vi "Multicolor_line_generator.vi"() -> ()   [LabVIEW 2020]
uses:
  ASLM project/type_defs/Laser_toggles_typedef.ctl
  <vilib>/Utility/file.llb/Read Delimited Spreadsheet (DBL).vi
  <vilib>/measure/NI_MABase.lvlib
panel:
  in  "Laser 642 nm power":dbl(slide) min=0.0 max=5.0 scale=0.0..5.0
  in  "Laser 595 nm power":dbl(slide) min=0.0 max=5.0 scale=0.0..5.0
  in  "Laser 560 nm power":dbl(slide) min=0.0 max=5.0 scale=0.0..5.0
  in  "Laser 488 nm power":dbl(slide) min=0.0 max=5.0 scale=0.0..5.0
  in  "Time for one frame":dbl
  out "Number of active lasers":dbl
  out "Laser Toggles":T1
  in  "Time between acquisitions":dbl
  in  "File to read":path=path "C:/Users/Hannah/Downloads/newcalibration_voice coil input_25msflyback_3075datapoints.txt"
  out "LabVIEW generated Sawtooth input (blue) and Camera trigger (red)":waveform(dbl)[](graph)=[{"t0"=timestamp(0 s since 1904-01-01), "dt"=1.0, "Y"=array[3075 elements]}, {"t0"=timestamp(0 s since 1904-01-01), "dt"=0.001, "Y"=array[3075 elements]}, {"t0"=timestamp(0 s since 1904-01-01), "dt"=0.001, "Y"=array[3075 elements]}, {"t0"=timestamp(0 s since 1904-01-01), "dt"=0.001, "Y"=array[3075 elements]}]
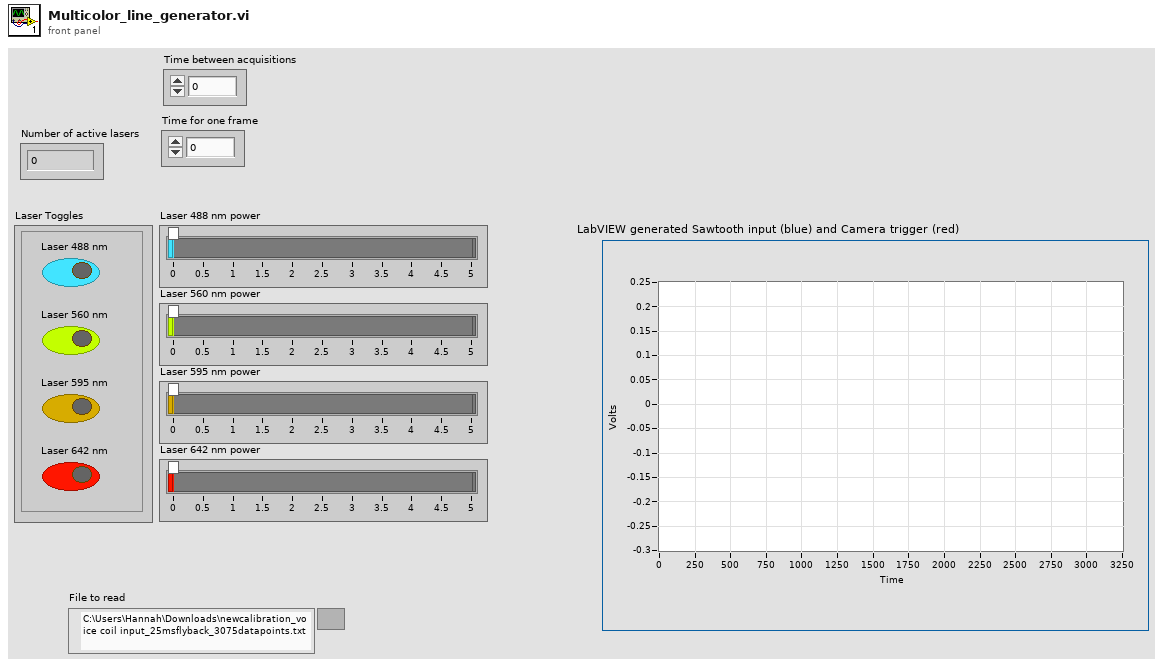
[diagram p1: front panel]
types:
  T1 = typedef "Laser_toggles_typedef.ctl" = cluster{"Laser 488 nm":bool, "Laser 560 nm":bool, "Laser 595 nm":bool, "Laser 642 nm":bool}
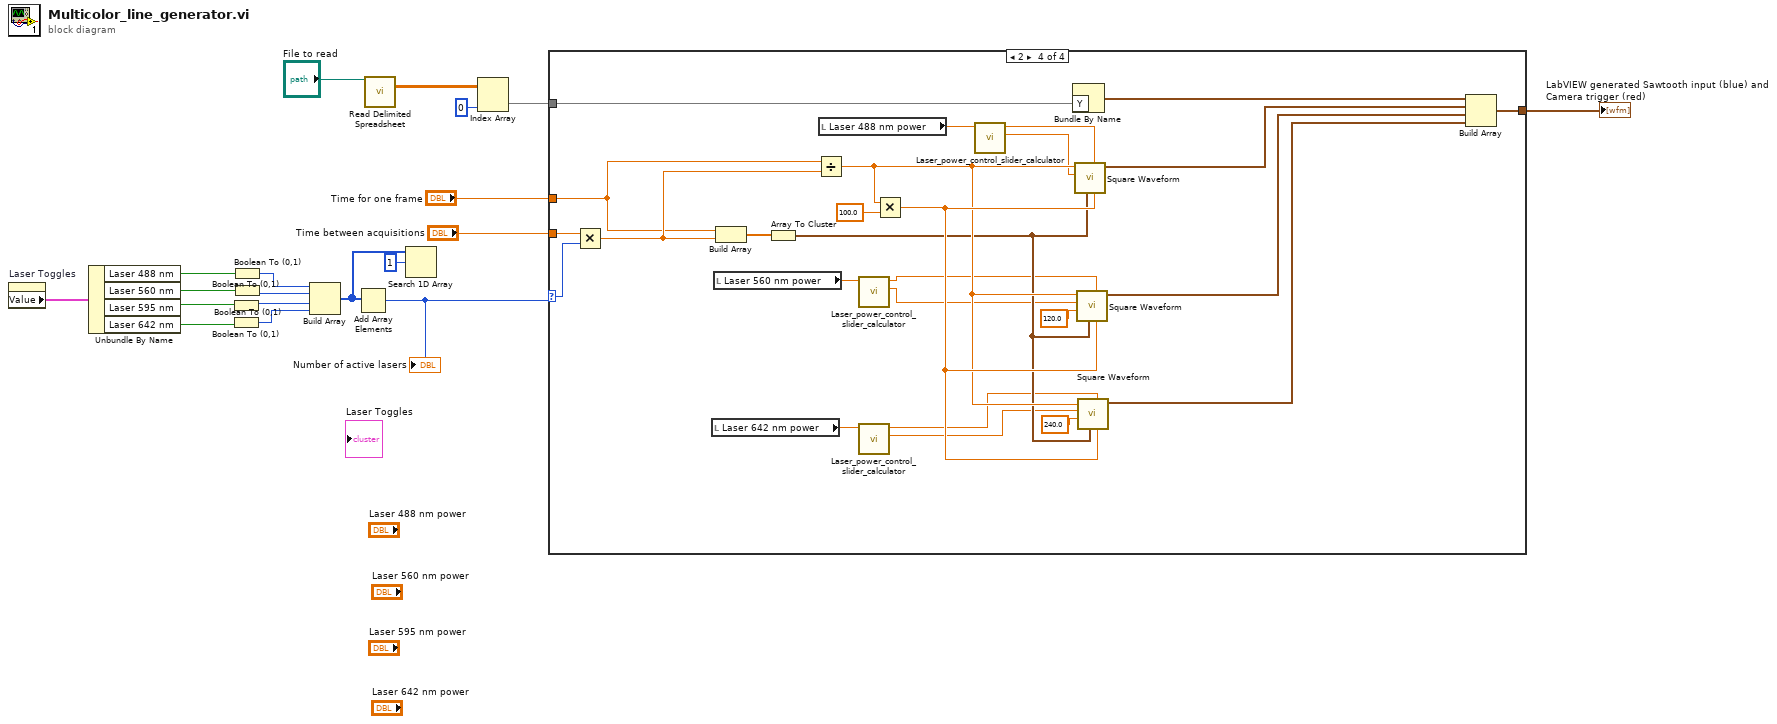
[diagram p0: block diagram]
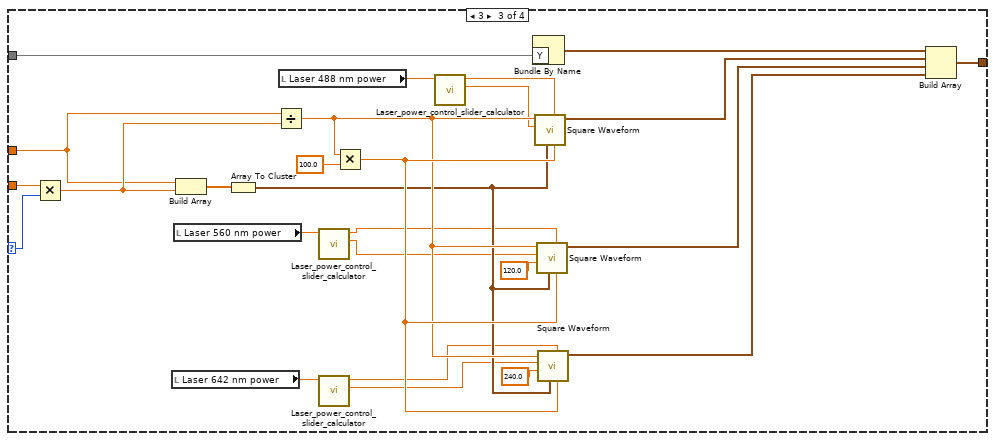
[diagram p4: hidden frame]
diagram:
  n1 = property on="Laser Toggles" class="Clust (strict)"() -> ("Value"=w14:T1)  [unwired: 2 in, 2 out]
  n2 = Unbundle By Name(w14) -> ("Laser 488 nm"=w13:bool, "Laser 560 nm"=w12:bool, "Laser 595 nm"=w10:bool, "Laser 642 nm"=w11:bool)
  n3 = Boolean To (0,1)(Boolean=w10) -> (0, 1=w7:i16)
  n4 = Boolean To (0,1)(Boolean=w11) -> (0, 1=w6:i16)
  n5 = Boolean To (0,1)(Boolean=w13) -> (0, 1=w9:i16)
  n6 = Boolean To (0,1)(Boolean=w12) -> (0, 1=w8:i16)
  n7 = Build Array(w9, w8, w7, w6) -> (w2:i16[])
  n8 = Add Array Elements(numeric array=w2) -> (sum=w5:i16)
  "Number of active lasers" <- w5
  n9 = call-poly <vilib>:"Read Delimited Spreadsheet.vi"("file path (dialog if empty)"="File to read") -> ("all rows"=w18:dbl[][])  [unwired: 9 in, 5 out]
  n10 = Search 1D Array(1D array=w2, element=i16 1) -> ()  [unwired: 1 in, 1 out]
  n11 = Index Array(array=w18, index (col)=0 ("disabled index (col)")) -> (element=w16:dbl[])  [unwired: 1 in]
  n12 = case shown="2" w5 {
    selector: w5 -> [_ _ w34 w60]
    tunnel: w16 -> [_ _ w36 w62]
    tunnel: [_ _ w35 w61] -> w15
    tunnel: "Time between acquisitions" -> [_ _ w33 w59]
    tunnel: "Time for one frame" -> [_ _ w30 w56]
    frame 0, Default {
    }
    frame 1 {
    }
    frame 3 {
      n13 = Multiply(x=w33, y=w34) -> (x*y=w32:dbl)
      n14 = local read "Laser 642 nm power"() -> (w22:dbl)
      n15 = local read "Laser 560 nm power"() -> (w25:dbl)
      n16 = Build Array(w30, w32) -> (w29:dbl[])
      n17 = Array To Cluster(array=w29) -> (cluster=w31:cluster{"[0]":dbl, "[1]":dbl})
      n18 = Divide(x=w30, y=w32) -> (x/y=w37:dbl)
      n19 = local read "Laser 488 nm power"() -> (w28:dbl)
      n20 = call "Laser_power_control_slider_calculator.vi"("Laser 488 nm power"=w25) -> ("Amplitude"=w23:dbl, "Offset"=w24:dbl)  [unwired: 9 in]
      n21 = call "Laser_power_control_slider_calculator.vi"("Laser 488 nm power"=w22) -> ("Amplitude"=w20:dbl, "Offset"=w21:dbl)  [unwired: 9 in]
      n22 = Multiply(x=w37, y=100.0) -> (x*y=w39:dbl)
      n23 = call "Laser_power_control_slider_calculator.vi"("Laser 488 nm power"=w28) -> ("Amplitude"=w26:dbl, "Offset"=w27:dbl)  [unwired: 9 in]
      n24 = Bundle By Name("Y"=w36) -> (w41:waveform(dbl))  [unwired: 1 in]
      n25 = call <vilib>:"Square Waveform.vi"("duty cycle (%)"=w39, "offset"=w27, "sampling info"=w31, "amplitude"=w26, "frequency"=w37) -> ("signal out"=w45:waveform(dbl))  [unwired: 5 in, 1 out]
      n26 = call <vilib>:"Square Waveform.vi"("duty cycle (%)"=w39, "offset"=w24, "sampling info"=w31, "phase"=120.0, "amplitude"=w23, "frequency"=w37) -> ("signal out"=w44:waveform(dbl))  [unwired: 4 in, 1 out]
      n27 = call <vilib>:"Square Waveform.vi"("duty cycle (%)"=w39, "offset"=w21, "sampling info"=w31, "phase"=240.0, "amplitude"=w20, "frequency"=w37) -> ("signal out"=w43:waveform(dbl))  [unwired: 4 in, 1 out]
      n28 = Build Array(w41, w45, w44, w43) -> (w35:waveform(dbl)[])
    }
    frame 2 {
      n29 = Multiply(x=w59, y=w60) -> (x*y=w58:dbl)
      n30 = local read "Laser 642 nm power"() -> (w48:dbl)
      n31 = local read "Laser 560 nm power"() -> (w51:dbl)
      n32 = Build Array(w56, w58) -> (w55:dbl[])
      n33 = Array To Cluster(array=w55) -> (cluster=w57:cluster{"[0]":dbl, "[1]":dbl})
      n34 = Divide(x=w56, y=w58) -> (x/y=w63:dbl)
      n35 = local read "Laser 488 nm power"() -> (w54:dbl)
      n36 = call "Laser_power_control_slider_calculator.vi"("Laser 488 nm power"=w51) -> ("Amplitude"=w49:dbl, "Offset"=w50:dbl)  [unwired: 9 in]
      n37 = call "Laser_power_control_slider_calculator.vi"("Laser 488 nm power"=w48) -> ("Amplitude"=w46:dbl, "Offset"=w47:dbl)  [unwired: 9 in]
      n38 = Multiply(x=w63, y=100.0) -> (x*y=w65:dbl)
      n39 = call "Laser_power_control_slider_calculator.vi"("Laser 488 nm power"=w54) -> ("Amplitude"=w52:dbl, "Offset"=w53:dbl)  [unwired: 9 in]
      n40 = Bundle By Name("Y"=w62) -> (w67:waveform(dbl))  [unwired: 1 in]
      n41 = call <vilib>:"Square Waveform.vi"("duty cycle (%)"=w65, "offset"=w53, "sampling info"=w57, "amplitude"=w52, "frequency"=w63) -> ("signal out"=w71:waveform(dbl))  [unwired: 5 in, 1 out]
      n42 = call <vilib>:"Square Waveform.vi"("duty cycle (%)"=w65, "offset"=w50, "sampling info"=w57, "phase"=120.0, "amplitude"=w49, "frequency"=w63) -> ("signal out"=w70:waveform(dbl))  [unwired: 4 in, 1 out]
      n43 = call <vilib>:"Square Waveform.vi"("duty cycle (%)"=w65, "offset"=w47, "sampling info"=w57, "phase"=240.0, "amplitude"=w46, "frequency"=w63) -> ("signal out"=w69:waveform(dbl))  [unwired: 4 in, 1 out]
      n44 = Build Array(w67, w71, w70, w69) -> (w61:waveform(dbl)[])
    }
  }
  "LabVIEW generated Sawtooth input (blue) and Camera trigger (red)" <- w15
